vi "Get RS485 Address.vi"(4 "error in":errorcluster, 7 "VISA resource name in":refnum<visa-resource-name>) -> (0 "Fehler (Ausgang)":errorcluster, 1 "RS485-Address":u8, 3 "VISA resource name out":refnum<visa-resource-name>)   [LabVIEW 2018, in "JULABO DeviceDriver.lvlib"]
doc: "This VI returns the adjusted RS485 address."
uses:
  JULABO DeviceDriver.lvlib
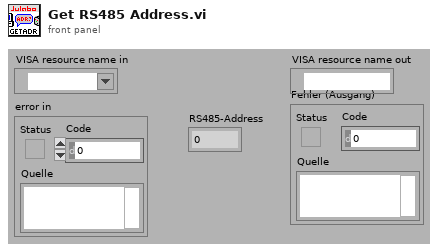
[diagram p1: front panel]
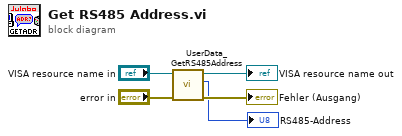
[diagram p0: block diagram]
diagram:
  n1 = call "UserData_GetRS485Address.vi"("Fehler (Eingang)"="error in", "VISA resource name in"="VISA resource name in") -> ("Fehler (Ausgang)"=→"Fehler (Ausgang)":errorcluster, "Address"=→"RS485-Address":u8, "VISA resource name out"=→"VISA resource name out":refnum<visa-resource-name>)  [unwired: 3 in]
